vi "Save.vi"(8 "error in":errorcluster, 11 "state in":T1) -> (0 "error out":errorcluster, 3 "state out":T1)   [LabVIEW 2013]
uses:
  Controls/StateCluster.ctl
  CEF_TreeControl/Repository/NISE_CEF_Repository.lvclass
  CEF_TreeControl/Node/NodeRef.ctl
  CEF_TreeControl/Node/NISE_CEF_Node.lvclass
  CEF_TreeControl/Node/UserEventRef.ctl
  CEF_TreeControl/Controls/EventCluster.ctl
  CEF_TreeControl/NISE_CEF_TreeControl.lvlib
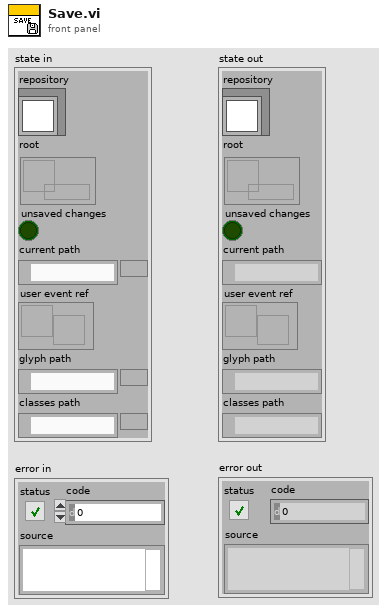
[diagram p1: front panel]
types:
  T1 = typedef "StateCluster.ctl" = cluster{"repository":refnum<class "NISE_CEF_Repository.lvclass">, "root":T2, "unsaved changes":bool, "current path":path, "user event ref":T3, "glyph path":path, "classes path":path}
  T2 = typedef "NISE_CEF_Node.lvclass/NodeRef.ctl" = refnum<data-value>
  T3 = typedef "NISE_CEF_Node.lvclass/UserEventRef.ctl" = refnum<user-event>
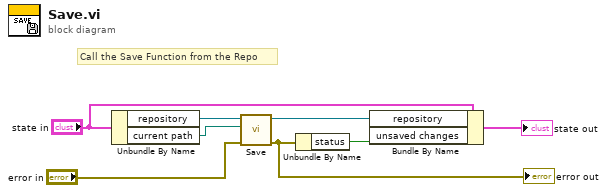
[diagram p0: block diagram]
diagram:
  # "Call the Save Function from the Repo"
  n1 = Unbundle By Name("state in") -> ("repository"=w8:refnum<class "NISE_CEF_Repository.lvclass">, "current path"=w2:path)
  n2 = call-dynamic "Save.vi"("error in"="error in", "file path"=w2, "repository in"=w8) -> ("error out"=w4:errorcluster, "repository out"=w1:refnum<class "NISE_CEF_Repository.lvclass">)  [unwired: 7 in]
  "error out" <- w4
  n3 = Unbundle By Name(w4) -> ("status"=w3:bool)
  n4 = Bundle By Name(cluster="state in", "repository"=w1, "unsaved changes"=w3) -> (→"state out":T1)
